vi "Bellows Tune.vi"(0 "Tune Amount":i32) -> ()   [LabVIEW 2019]
uses:
  MWC Global.vi
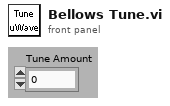
[diagram p1: front panel]
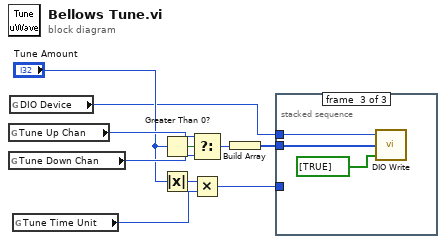
[diagram p0: block diagram]
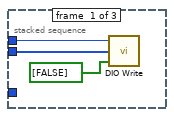
[diagram p2: hidden frame]
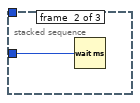
[diagram p3: hidden frame]
diagram:
  n1 = global read "MWC Global.vi" "Tune Up Chan"() -> (w8:i32)
  n2 = global read "MWC Global.vi" "Tune Down Chan"() -> (w9:i32)
  n3 = global read "MWC Global.vi" "DIO Device"() -> (w4:i32)
  n4 = global read "MWC Global.vi" "Tune Time Unit"() -> (w5:i32)
  n5 = Greater Than 0?(x="Tune Amount") -> (x > 0?=w10:bool)
  n6 = Absolute Value(x="Tune Amount") -> (abs(x)=w6:i32)
  n7 = Select(t=w8, s=w10, f=w9) -> (s? t:f=w3:i32)
  n8 = Multiply(x=w6, y=w5) -> (x*y=w1:i32)
  n9 = Build Array(w3) -> (w2:i32[])
  n10 = stacked-sequence {
    tunnel: w4 -> [w13 _ w17]
    tunnel: w2 -> [w12 _ w16]
    tunnel: w1 -> [_ w14 _]
    frame #0 {
      n11 = call "DIO Write.vi"("Data"=bool[] [FALSE], "Channels"=w12, "device"=w13) -> ()  [unwired: 1 out]
    }
    frame #1 {
      n12 = Wait (ms)(milliseconds to wait=w14) -> ()  [unwired: 1 out]
    }
    frame #2 {
      n13 = call "DIO Write.vi"("Data"=bool[] [TRUE], "Channels"=w16, "device"=w17) -> ()  [unwired: 1 out]
    }
  }
